vi "studio.vi"() -> ()   [LabVIEW 2017]
uses:
  <vilib>/sound2/lvsound2.llb/Sound Data Format.ctl
  <vilib>/sound2/lvsound2.llb/Sampling Mode.ctl
  <vilib>/Analysis/3filter.llb/Filter Passband Type.ctl
  <vilib>/sound2/lvsound2.llb/Sound File Info (path).vi
  <vilib>/Analysis/3filter.llb/Butterworth Filter (DBL).vi
  <vilib>/sound2/lvsound2.llb/Sound Output Set Volume (Single).vi
  <vilib>/sound2/lvsound2.llb/Sound Output Write (DBL Single).vi
  <vilib>/sound2/lvsound2.llb/Sound Input Read (DBL).vi
  <vilib>/Analysis/NI_AALBase.lvlib
panel:
  in  "low cutoff freq: fl":dbl=0.12500000000000006 format="%0.4f"
  in  "high cutoff freq: fh":dbl=0.45000000000000007
  out "Modified Waveform":waveform(dbl)(graph)
  in  "Volume":dbl(knob) scale=0.0..100.0
  in  "Output File":path
  out "Sound Format":T1={"sample rate (S/s)"=44100.0, "number of channels"=2, "bits per sample"=16}
  in  "Mode":T2(ring)=enum."Records Audio "
  out "sound format 2":T1={"sample rate (S/s)"=22050.0, "number of channels"=2, "bits per sample"=16}
  out "Input Audio":waveform(dbl)(graph)
  in  "File Path Control":path=path "/Users/Tony/Desktop/LabVIEW/sample_audio.wav"
  out "Recorded  Audio":waveform(dbl)[](graph)
  in  "Number of Samples/ch":i32=10000
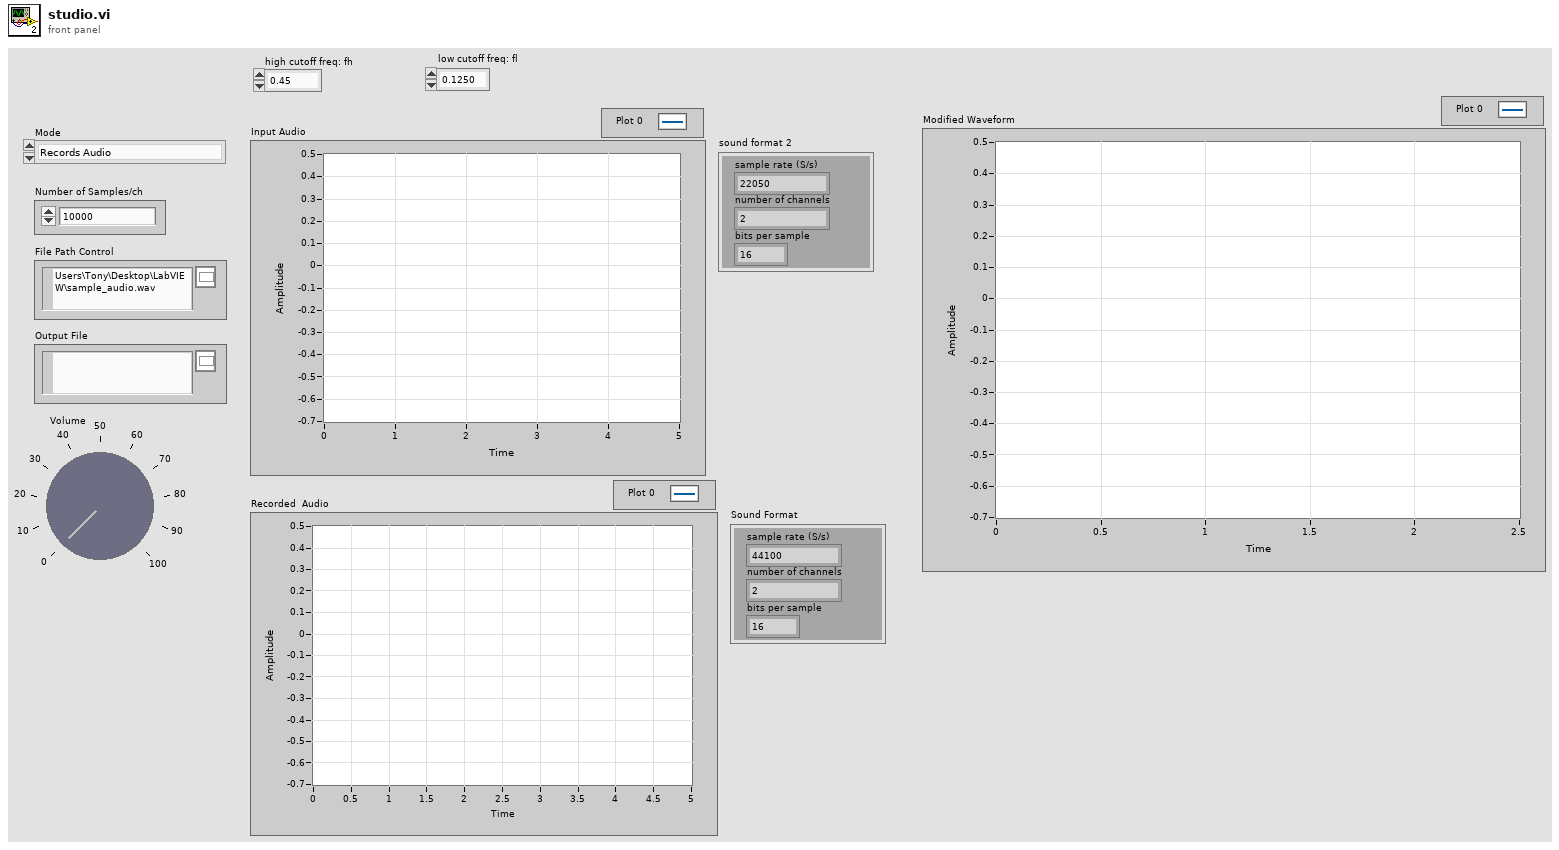
[diagram p1: front panel]
types:
  T1 = typedef "Sound Data Format.ctl" = cluster{"sample rate (S/s)":dbl, "number of channels":i32, "bits per sample":i32}
  T2 = enum16{"Open Audio File", "Records Audio ", "Reverse", "Slow Down", "Speeds Up", "High Pass Filter", "Low Pass Filter", "Saves Processed Audio"}
  T3 = typedef "NI_AALBase.lvlib/Filter Passband Type.ctl" = enum32{"Lowpass", "Highpass", "Bandpass", "Bandstop"}
  T4 = typedef "Sampling Mode.ctl" = i32
  T5 = typedef "Sound Input Task ID.ctl" = u32
  T6 = typedef "Sound Output Task ID.ctl" = u32
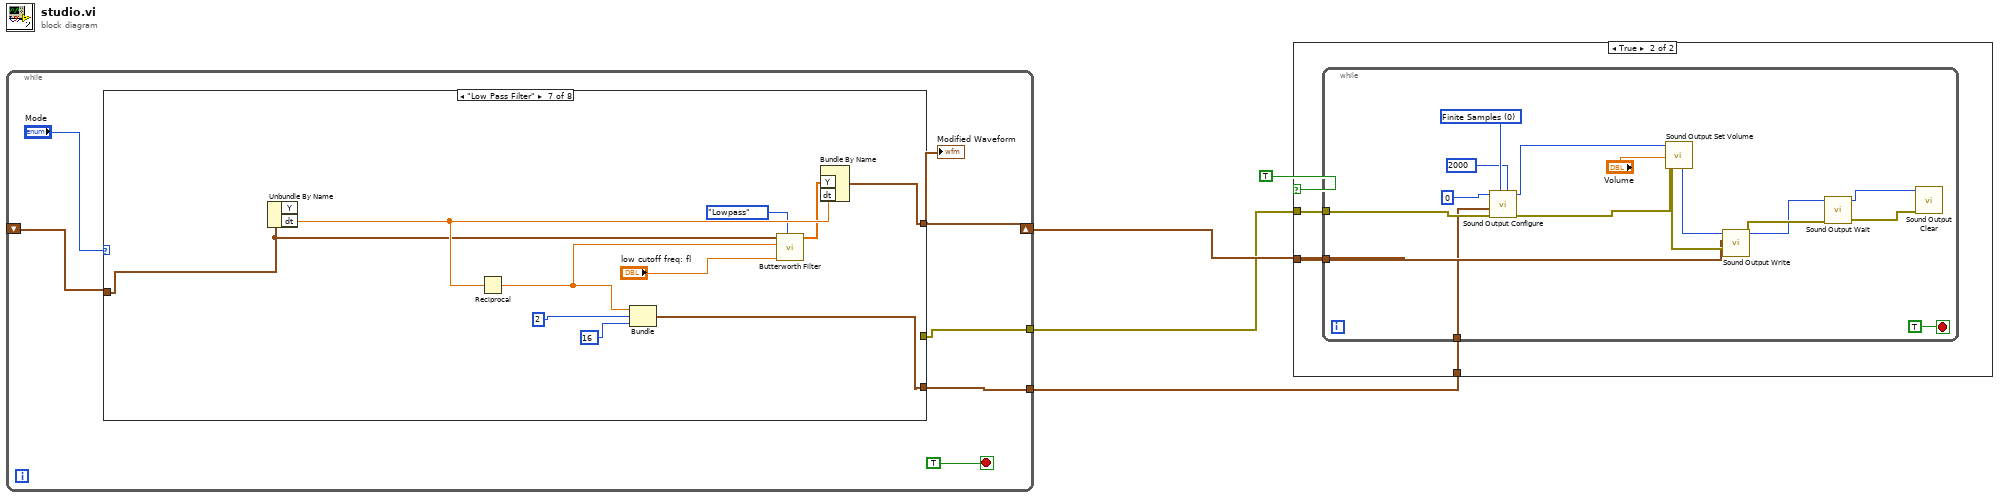
[diagram p0: block diagram]
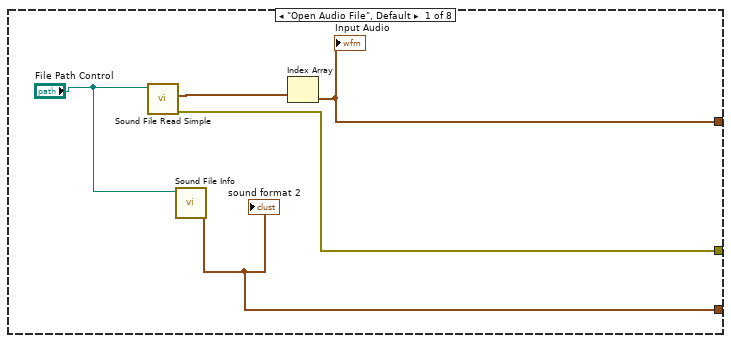
[diagram p3: hidden frame]
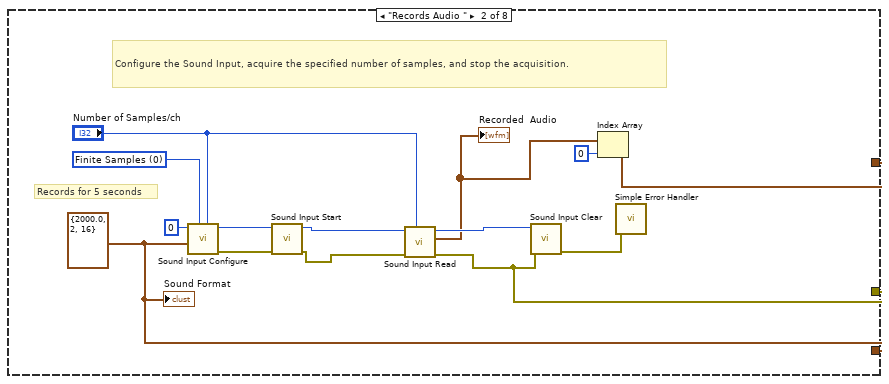
[diagram p4: hidden frame]
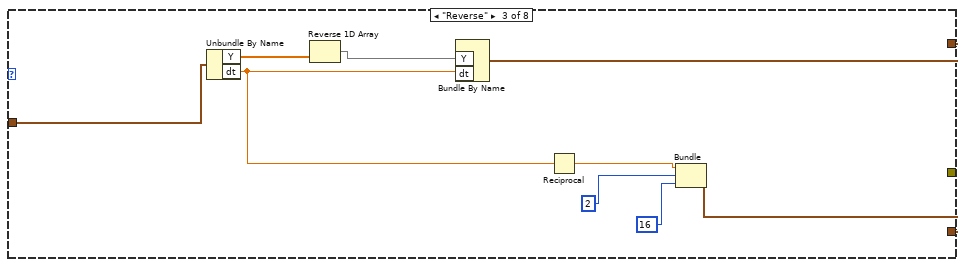
[diagram p5: hidden frame]
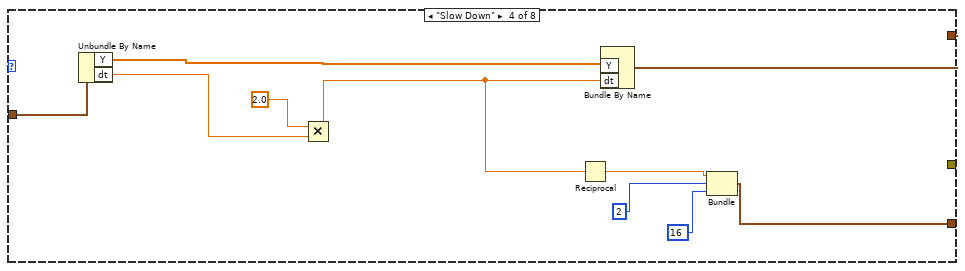
[diagram p6: hidden frame]
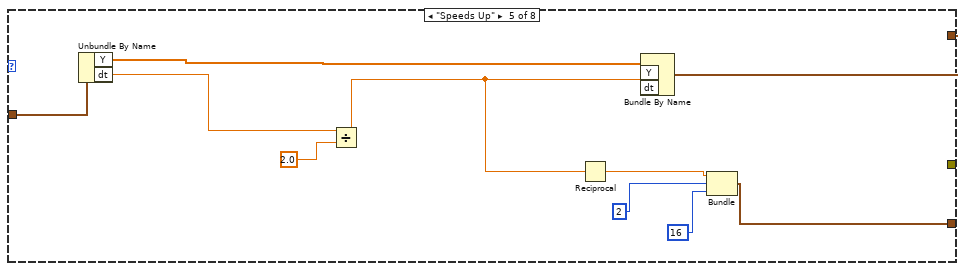
[diagram p7: hidden frame]
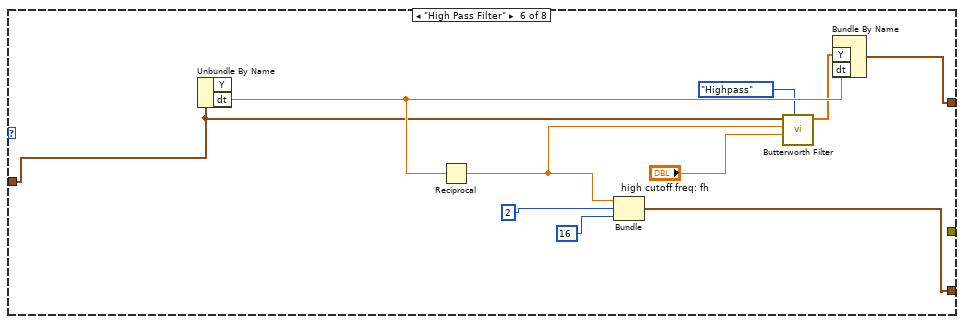
[diagram p8: hidden frame]
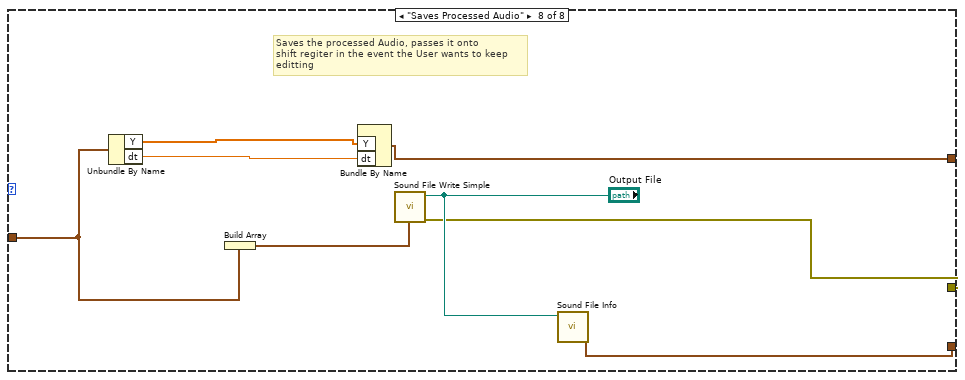
[diagram p9: hidden frame]
diagram:
  n1 = while {
    shift-right: [w5] -> w3
    shift-left: _ -> [w10]
    tunnel: [w9] -> w2
    tunnel: [w8] -> w1
    stop <- TRUE stop-if-true
    n2 = case shown="\"Low Pass Filter\"" "Mode" {
      tunnel: w10 -> [_ _ w37 w46 w57 w62 w73 w81]
      tunnel: [w13 w16 w30 w44 w56 w60 w71 w80] -> w5
      tunnel: [w12 w18 _ _ _ _ _ w84] -> w9
      tunnel: [w11 w17 w33 w39 w51 w59 w70 w85] -> w8
      frame "Open Audio File", Default {
        n3 = call <vilib>:"Sound File Read Simple.vi"("path"="File Path Control") -> ("error out"=w12:errorcluster, "data"=w15:waveform(dbl)[])  [unwired: 7 in, 2 out]
        n4 = call-poly <vilib>:"Sound File Info.vi"("path"="File Path Control") -> ("sound format"=w11:T1)  [unwired: 7 in, 3 out]
        "sound format 2" <- w11
        n5 = Index Array(array=w15) -> (element=w13:waveform(dbl))  [unwired: 1 in]
        "Input Audio" <- w13
      }
      frame "Records Audio " {
        w17 = T1 {"sample rate (S/s)"=2000.0, "number of channels"=2, "bits per sample"=16} ("Sound Format")
        w29 = T4 0 items=["Finite Samples", "Continuous Samples"] ("sample mode")
        # "Records for 5 seconds"
        # "Configure the Sound Input, acquire the specified number of samples, and stop the acquisition."
        n6 = call <vilib>:"Sound Input Configure.vi"("number of samples/ch"="Number of Samples/ch", "sample mode"=w29, "sound format"=w17, "device ID"=u32 0) -> ("error out"=w24:errorcluster, "task ID"=w23:T5)  [unwired: 6 in]
        n7 = call <vilib>:"Sound Input Start.vi"("error in (no error)"=w24, "task ID"=w23) -> ("error out"=w25:errorcluster, "task ID out"=w26:T5)  [unwired: 8 in]
        n8 = call-poly <vilib>:"Sound Input Read.vi"("number of samples/ch"="Number of Samples/ch", "error in (no error)"=w25, "task ID"=w26) -> ("error out"=w18:errorcluster, "data"=w20:waveform(dbl)[], "task ID out"=w21:T5)  [unwired: 6 in]
        "Recorded  Audio" <- w20
        n9 = call <vilib>:"Sound Input Clear.vi"("error in (no error)"=w18, "task ID"=w21) -> ("error out"=w27:errorcluster)  [unwired: 9 in]
        n10 = Index Array(array=w20, index=0) -> (element=w16:waveform(dbl))
        n11 = call <vilib>:"Simple Error Handler.vi"("error in (no error)"=w27) -> ()  [unwired: 4 in, 5 out]
        "Sound Format" <- w17
      }
      frame "Reverse" {
        n12 = Unbundle By Name(w37) -> ("Y"=w38:dbl[], "dt"=w31:dbl)
        n13 = Reverse 1D Array(array=w38) -> (reversed array=w32:dbl[])
        n14 = Bundle By Name("Y"=w32, "dt"=w31) -> (w30:waveform(dbl))  [unwired: 1 in]
        n15 = Reciprocal(x=w31) -> (1/x=w36:dbl)
        n16 = Bundle(w36, 2, 16) -> (w33:cluster{dbl, i32, i32})  [unwired: 1 in]
      }
      frame "Slow Down" {
        n17 = Unbundle By Name(w46) -> ("Y"=w47:dbl[], "dt"=w48:dbl)
        n18 = Multiply(x=2.0, y=w48) -> (x*y=w40:dbl)
        n19 = Reciprocal(x=w40) -> (1/x=w43:dbl)
        n20 = Bundle By Name("Y"=w47, "dt"=w40) -> (w44:waveform(dbl))  [unwired: 1 in]
        n21 = Bundle(w43, 2, 16) -> (w39:cluster{dbl, i32, i32})  [unwired: 1 in]
      }
      frame "Speeds Up" {
        n22 = Unbundle By Name(w57) -> ("Y"=w58:dbl[], "dt"=w50:dbl)
        n23 = Divide(x=w50, y=2.0) -> (x/y=w52:dbl)
        n24 = Reciprocal(x=w52) -> (1/x=w55:dbl)
        n25 = Bundle By Name("Y"=w58, "dt"=w52) -> (w56:waveform(dbl))  [unwired: 1 in]
        n26 = Bundle(w55, 2, 16) -> (w51:cluster{dbl, i32, i32})  [unwired: 1 in]
      }
      frame "High Pass Filter" {
        n27 = Unbundle By Name(w62) -> ("dt"=w66:dbl)  [unwired: 1 out]
        n28 = Reciprocal(x=w66) -> (1/x=w63:dbl)
        n29 = Bundle(w63, 2, 16) -> (w59:cluster{dbl, i32, i32})  [unwired: 1 in]
        n30 = call-poly <vilib>:"Butterworth Filter.vi"("filter type"=Filter_Passband_Type."Highpass", "high cutoff freq: fh"="high cutoff freq: fh", "sampling freq: fs"=w63, "X"=w62) -> ("Filtered X"=w61:dbl[])  [unwired: 4 in, 1 out]
        n31 = Bundle By Name("Y"=w61, "dt"=w66) -> (w60:waveform(dbl))  [unwired: 1 in]
      }
      frame "Low Pass Filter" {
        n32 = Unbundle By Name(w73) -> ("dt"=w76:dbl)  [unwired: 1 out]
        n33 = Reciprocal(x=w76) -> (1/x=w74:dbl)
        n34 = Bundle(w74, 2, 16) -> (w70:cluster{dbl, i32, i32})  [unwired: 1 in]
        n35 = call-poly <vilib>:"Butterworth Filter.vi"("filter type"=Filter_Passband_Type."Lowpass", "low cutoff freq: fl"="low cutoff freq: fl", "sampling freq: fs"=w74, "X"=w73) -> ("Filtered X"=w72:dbl[])  [unwired: 4 in, 1 out]
        n36 = Bundle By Name("Y"=w72, "dt"=w76) -> (w71:waveform(dbl))  [unwired: 1 in]
      }
      frame "Saves Processed Audio" {
        # "Saves the processed Audio, passes it onto\nshift regiter in the event the User wants to keep\neditting"
        n37 = Unbundle By Name(w81) -> ("Y"=w82:dbl[], "dt"=w83:dbl)
        n38 = Build Array(w81) -> (w79:waveform(dbl)[])
        n39 = Bundle By Name("Y"=w82, "dt"=w83) -> (w80:waveform(dbl))  [unwired: 1 in]
        n40 = call <vilib>:"Sound File Write Simple.vi"("data"=w79, "path"="Output File") -> ("error out"=w84:errorcluster)  [unwired: 8 in, 1 out]
        n41 = call-poly <vilib>:"Sound File Info.vi"("path"="Output File") -> ("sound format"=w85:T1)  [unwired: 7 in, 3 out]
      }
    }
    "Modified Waveform" <- w5
  }
  n42 = case shown="True" TRUE {
    tunnel: w3 -> [_ w89]
    tunnel: w2 -> [_ w88]
    tunnel: w1 -> [_ w87]
    frame False {
    }
    frame True {
      n43 = while {
        tunnel: w89 -> [w95]
        tunnel: w88 -> [w94]
        tunnel: w87 -> [w93]
        stop <- TRUE stop-if-true
        w105 = T4 0 items=["Finite Samples", "Continuous Samples"] ("sample mode")
        n44 = call <vilib>:"Sound Output Configure.vi"("number of samples/ch"=2000, "sample mode"=w105, "error in (no error)"=w94, "sound format"=w93, "device ID"=u32 0) -> ("error out"=w102:errorcluster, "task ID"=w103:T6)  [unwired: 5 in]
        n45 = call-poly <vilib>:"Sound Output Set Volume.vi"("error in (no error)"=w102, "volume"="Volume", "task ID"=w103) -> ("error out"=w100:errorcluster, "task ID out"=w101:T6)  [unwired: 7 in]
        n46 = call-poly <vilib>:"Sound Output Write.vi"("error in (no error)"=w100, "data"=w95, "task ID"=w101) -> ("error out"=w99:errorcluster, "task ID out"=w98:T6)  [unwired: 7 in]
        n47 = call <vilib>:"Sound Output Wait.vi"("error in (no error)"=w99, "task ID"=w98) -> ("error out"=w96:errorcluster, "task ID out"=w97:T6)  [unwired: 8 in]
        n48 = call <vilib>:"Sound Output Clear.vi"("error in (no error)"=w96, "task ID"=w97) -> ()  [unwired: 9 in, 1 out]
      }
    }
  }
